vi "Shutdown.vi"(8 "error in":errorcluster, 10 "Boiler Controls":T1 {"Fuel Valve Position" min=0.0 max=100.0 scale=0.0..100.0 scale format="%.2f"}, 11 "Boiler Simulation Controls":T2 {"Flame Sensor Value (%)" min=0.0 max=100.0 scale=0.0..100.0}) -> (0 "error out":errorcluster, 3 "shutdown":bool)   [LabVIEW 2015]
doc: "Generete true value if shutdown should occur. Conditions of shutdown are listed in specification."
uses:
  USB Template (LV 8.6)/Boiler/Controls/Boiler Simulation Controls.ctl
  USB Template (LV 8.6)/Boiler/Controls/Boiler Controls.ctl
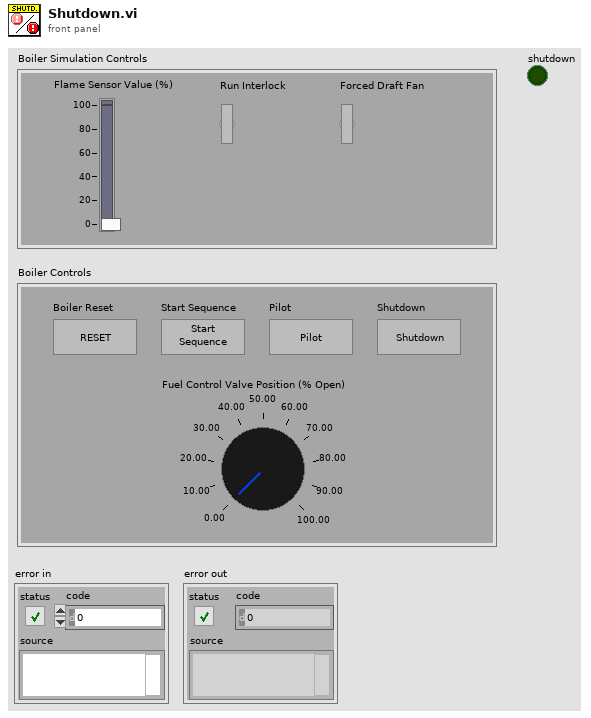
[diagram p1: front panel]
types:
  T1 = typedef "Boiler Controls.ctl" = cluster{"Boiler Reset":bool, "Start Sequence":bool, "Pilot":bool, "Shutdown":bool, "Fuel Valve Position":dbl}
  T2 = typedef "Boiler Simulation Controls.ctl" = cluster{"Flame Sensor Value (%)":dbl, "Run Interlock":bool, "Forced Draft Fan":bool}
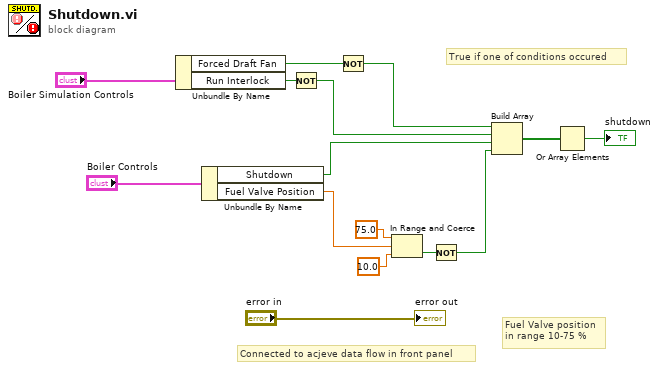
[diagram p0: block diagram]
diagram:
  # "True if one of conditions occured"
  # "Fuel Valve position\nin range 10-75 %"
  # "Connected to acjeve data flow in front panel"
  n1 = Unbundle By Name("Boiler Simulation Controls") -> ("Forced Draft Fan"=w10:bool, "Run Interlock"=w11:bool)
  n2 = Unbundle By Name("Boiler Controls") -> ("Shutdown"=w12:bool, "Fuel Valve Position"=w8:dbl)
  n3 = Not(x=w11) -> (.not. x?=w2:bool)
  n4 = Not(x=w10) -> (.not. x?=w1:bool)
  n5 = In Range and Coerce(upper limit=75.0, x=w8, lower limit=10.0) -> (In Range?=w9:bool)  [unwired: 1 out]
  n6 = Not(x=w9) -> (.not. x?=w13:bool)
  n7 = Build Array(w1, w2, w12, w13) -> (w14:bool[])
  n8 = Or Array Elements(Boolean array=w14) -> (logical OR=→"shutdown":bool)
  "error out" <- "error in"
